vi "setUp.vi"(8 "error in (no error)":errorcluster, 11 "reference in":refnum<class "Buffers Tests.lvclass">) -> (0 "error out":errorcluster, 3 "reference out":refnum<class "Buffers Tests.lvclass">)   [LabVIEW 2019, in "Buffers Tests.lvclass"]
doc: "setUp runs prior to the test method during test execution. Use this method to initialize any object data required by your tests."
uses:
  Buffers Tests.lvclass
  C:/Program Files (x86)/National Instruments/LabVIEW 2019/vi.lib/addons/_JKI Toolkits/VI Tester/TestCase.llb/TestCase.lvclass
  Buffers Tests.lvclass/Buffers Tests.ctl
  <vilib>/addons/_JKI Toolkits/VI Tester/TestCase.llb/TestCase.lvclass
  Classes/Buffers/Buffers.lvclass
  Classes/Buffer/Buffer.lvclass
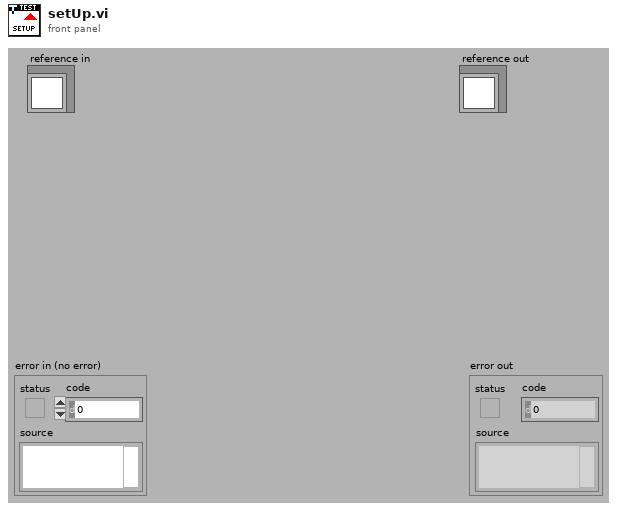
[diagram p1: front panel]
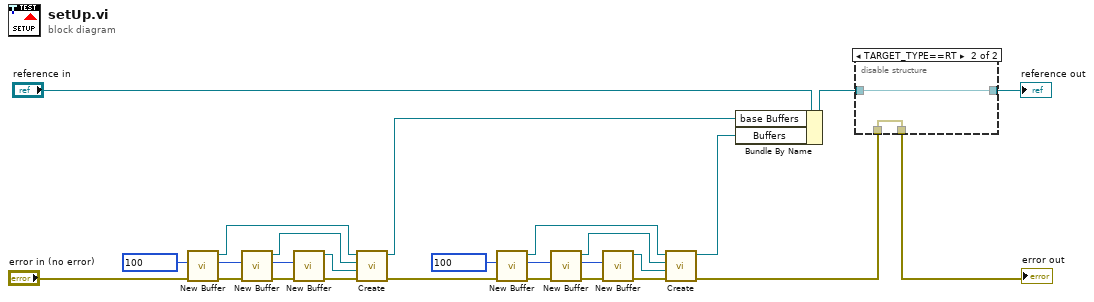
[diagram p0: block diagram]
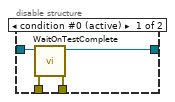
[diagram p2: hidden frame]
diagram:
  w8 = u64 100 ("buffer size")
  w15 = u64 100 ("buffer size")
  n1 = call "New Buffer.vi"("error in (no error)"="error in (no error)", "buffer size"=w15) -> ("error out"=w17:errorcluster, "Buffer out"=w14:refnum<class "Buffer.lvclass">)  [unwired: 8 in]
  n2 = call "New Buffer.vi"("error in (no error)"=w17, "buffer size"=w15) -> ("error out"=w16:errorcluster, "Buffer out"=w11:refnum<class "Buffer.lvclass">)  [unwired: 8 in]
  n3 = call "New Buffer.vi"("error in (no error)"=w16, "buffer size"=w15) -> ("error out"=w12:errorcluster, "Buffer out"=w13:refnum<class "Buffer.lvclass">)  [unwired: 8 in]
  n4 = call "Create.vi"("error in (no error)"=w12, "String Buffer (null)"=w13, "Async Buffer (null)"=w11, "Inline Buffer (null)"=w14) -> ("error out"=w3:errorcluster, "Buffers out"=w19:refnum<class "Buffers.lvclass">)  [unwired: 6 in]
  n5 = call "New Buffer.vi"("error in (no error)"=w3, "buffer size"=w8) -> ("error out"=w10:errorcluster, "Buffer out"=w7:refnum<class "Buffer.lvclass">)  [unwired: 8 in]
  n6 = call "New Buffer.vi"("error in (no error)"=w10, "buffer size"=w8) -> ("error out"=w9:errorcluster, "Buffer out"=w4:refnum<class "Buffer.lvclass">)  [unwired: 8 in]
  n7 = call "New Buffer.vi"("error in (no error)"=w9, "buffer size"=w8) -> ("error out"=w5:errorcluster, "Buffer out"=w6:refnum<class "Buffer.lvclass">)  [unwired: 8 in]
  n8 = call "Create.vi"("error in (no error)"=w5, "String Buffer (null)"=w6, "Async Buffer (null)"=w4, "Inline Buffer (null)"=w7) -> ("error out"=w2:errorcluster, "Buffers out"=w1:refnum<class "Buffers.lvclass">)  [unwired: 6 in]
  n9 = Bundle By Name(cluster="reference in", "base Buffers"=w19, "Buffers"=w1) -> (w21:refnum<class "Buffers Tests.lvclass">)
  n10 = disable-structure shown="TARGET_TYPE==RT" {
    disable-tunnel: w2 -> [w27 w28]
    disable-tunnel: [w26 w28] -> w23
    disable-tunnel: [w25 w29] -> w22
    disable-tunnel: w21 -> [w24 w29]
    frame condition #0 (active) {
      n11 = call <vilib>:"WaitOnTestComplete.vi"("error in (no error)"=w27, "TestCase in"=w24) -> ("error out"=w26:errorcluster, "TestCase out"=w25:refnum<class "Buffers Tests.lvclass">)  [unwired: 8 in]
    }
    frame condition #1 {
    }
  }
  "error out" <- w23
  "reference out" <- w22
